vi "Set LED power.vi"(8 "error in":errorcluster, 9 "LED Power (%)":dbl(slide) min=0.0 max=120.0 step=1.0 scale=0.0..100.0 scale format="%.1f", 10 "LED":enum8{"Red", "UV", "Green", "Blue"}(ring), 11 "LED handle in":refnum<visa-resource-name>) -> (0 "error out":errorcluster {"code" format="%.0x"}, 3 "LED handle out":refnum<visa-resource-name> caption="instrument handle out")   [LabVIEW 2017]
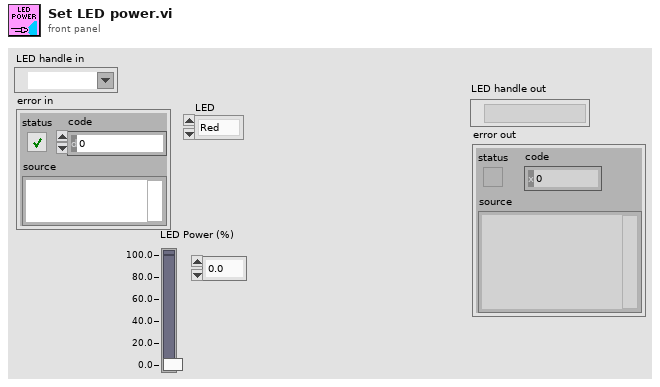
[diagram p1: front panel]
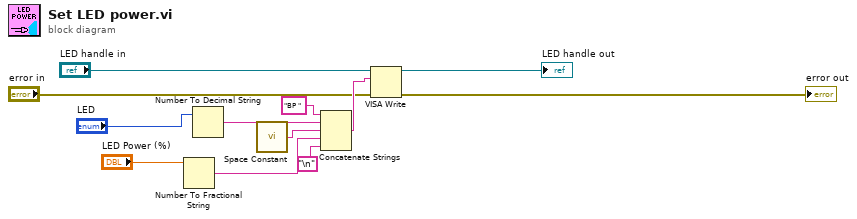
[diagram p0: block diagram]
diagram:
  n1 = Number To Fractional String(number="LED Power (%)") -> (F-format string=w5:string)  [unwired: 3 in]
  n2 = Number To Decimal String(number="LED") -> (decimal integer string=w2:string)  [unwired: 1 in]
  n3 = call <vilib>:"Space Constant.vi"() -> ("String"=w4:string)
  n4 = Concatenate Strings("BP " ("string"), w2, w4, w5, "\n") -> (w12:string)
  n5 = VISA Write(VISA resource name="LED handle in", write buffer=w12, error in (no error)="error in") -> (VISA resource name out=→"LED handle out":refnum<visa-resource-name>, error out=→"error out":errorcluster)  [unwired: 1 out]
